vi "TemperatureCorrection.vi"(0 "Action":enum16{"Reset", "Calculate", "Correct"}(ring), 1 "Sensor Index":i32, 2 "Current IN":dbl[](array[numeric]), 3 "Actual temperature":dbl, 4 "Correction temperature":dbl format="%.2f") -> (5 "Current OUT":dbl[](array[numeric]), 6 "Correction factor":dbl)   [LabVIEW 2013]
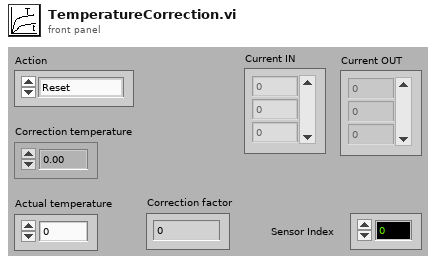
[diagram p1: front panel]
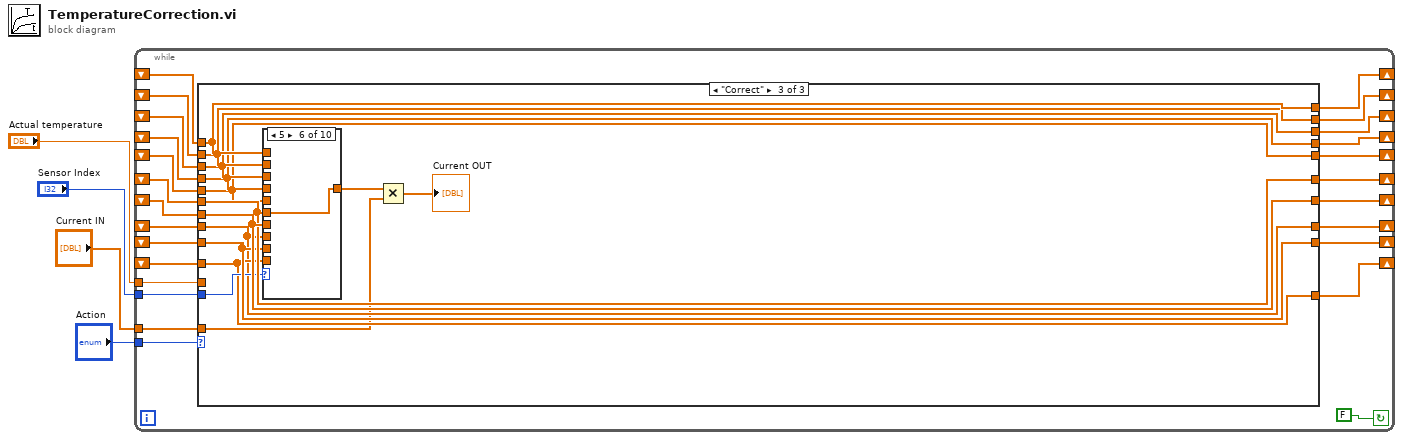
[diagram p0: block diagram]
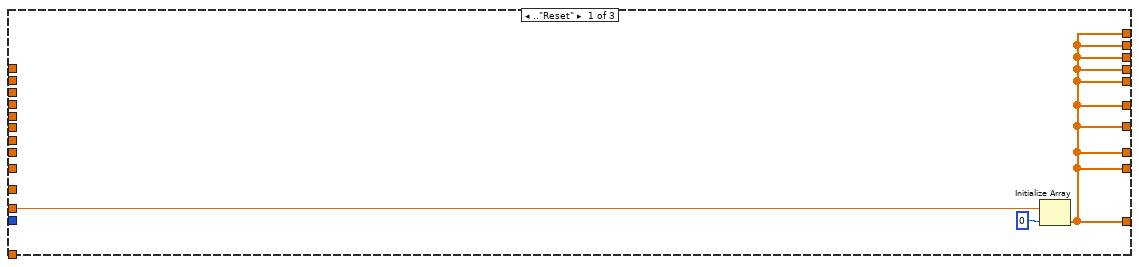
[diagram p2: hidden frame]
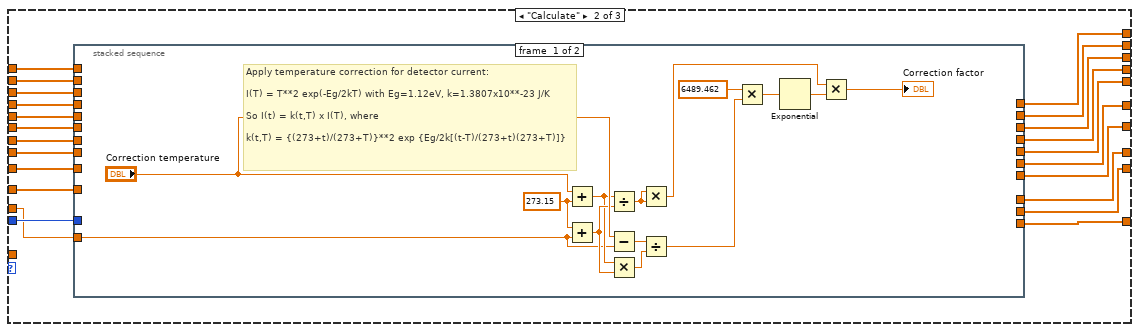
[diagram p3: hidden frame]
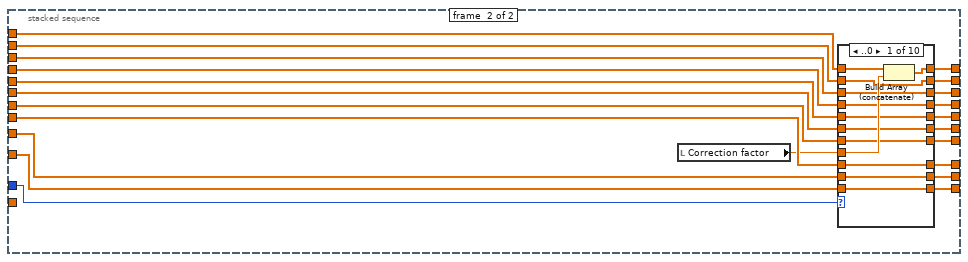
[diagram p4: hidden frame]
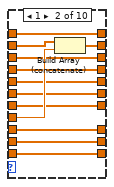
[diagram p5: hidden frame]
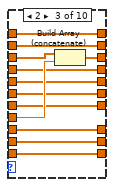
[diagram p6: hidden frame]
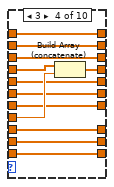
[diagram p7: hidden frame]
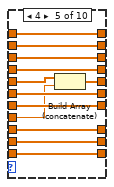
[diagram p8: hidden frame]
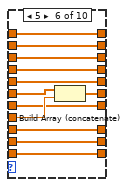
[diagram p9: hidden frame]
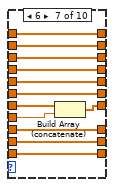
[diagram p10: hidden frame]
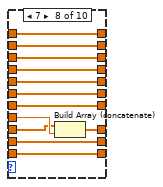
[diagram p11: hidden frame]
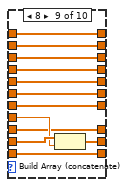
[diagram p12: hidden frame]
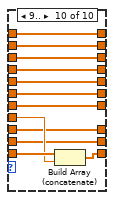
[diagram p13: hidden frame]
diagram:
  n1 = while {
    shift-left: _ -> [w10]
    shift-right: [w9] -> _
    tunnel: "Sensor Index" -> [w11]
    shift-left: _ -> [w12]
    shift-right: [w20] -> _
    shift-left: _ -> [w13]
    shift-right: [w8] -> _
    shift-left: _ -> [w14]
    shift-right: [w21] -> _
    shift-left: _ -> [w15]
    shift-right: [w22] -> _
    shift-left: _ -> [w16]
    shift-right: [w23] -> _
    shift-left: _ -> [w17]
    shift-right: [w24] -> _
    shift-left: _ -> [w18]
    shift-right: [w25] -> _
    shift-left: _ -> [w19]
    shift-right: [w26] -> _
    tunnel: "Actual temperature" -> [w28]
    shift-left: _ -> [w29]
    shift-right: [w27] -> _
    tunnel: "Current IN" -> [w6]
    tunnel: "Action" -> [w5]
    stop <- FALSE continue-if-true
    n2 = case shown="\"Correct\"" w5 {
      tunnel: [w32 w51 w224] -> w27
      tunnel: w29 -> [_ w53 w224]
      tunnel: w28 -> [w31 w52 _]
      tunnel: [w32 w49 w223] -> w26
      tunnel: [w32 w46 w222] -> w25
      tunnel: [w32 w45 w221] -> w24
      tunnel: [w32 w43 w220] -> w23
      tunnel: [w32 w42 w219] -> w22
      tunnel: [w32 w41 w218] -> w21
      tunnel: [w32 w40 w214] -> w8
      tunnel: [w32 w34 w217] -> w20
      tunnel: w19 -> [_ w50 w223]
      tunnel: w18 -> [_ w48 w222]
      tunnel: w17 -> [_ w47 w221]
      tunnel: w16 -> [_ w44 w220]
      tunnel: w15 -> [_ w39 w219]
      tunnel: w14 -> [_ w38 w218]
      tunnel: w13 -> [_ w37 w214]
      tunnel: w12 -> [_ w36 w217]
      tunnel: w11 -> [_ w54 w216]
      tunnel: w10 -> [_ w35 w215]
      tunnel: [w32 w33 w215] -> w9
      tunnel: w6 -> [_ _ w211]
      frame .."Reset" {
        n3 = Initialize Array(w31, 0) -> (w32:dbl[])
      }
      frame "Calculate" {
        n4 = stacked-sequence {
          tunnel: w54 -> [_ w90]
          tunnel: w53 -> [_ w89]
          tunnel: w52 -> [w55 _]
          tunnel: [_ w88] -> w51
          tunnel: w50 -> [_ w87]
          tunnel: [_ w86] -> w49
          tunnel: w48 -> [_ w85]
          tunnel: w47 -> [_ w84]
          tunnel: [_ w83] -> w46
          tunnel: [_ w82] -> w45
          tunnel: w44 -> [_ w81]
          tunnel: [_ w80] -> w43
          tunnel: [_ w79] -> w42
          tunnel: [_ w78] -> w41
          tunnel: [_ w77] -> w40
          tunnel: w39 -> [_ w76]
          tunnel: w38 -> [_ w75]
          tunnel: w37 -> [_ w74]
          tunnel: w36 -> [_ w73]
          tunnel: w35 -> [_ w72]
          tunnel: [_ w71] -> w34
          tunnel: [_ w70] -> w33
          frame #0 {
            w56 = 273.15
            # "Apply temperature correction for detector current:\n\nI(T) = T**2 exp(-Eg/2kT) with Eg=1.12eV, k=1.3807x10**-23 J/K\n\nSo I(t) = k(t,T) x I(T), where\n\nk(t,T) = {(273+t)/(273+T)}**2 exp {Eg/2k[(t-T)/(273+t)(273+T)]}"
            n5 = Add(x="Correction temperature", y=w56) -> (x+y=w58:dbl)
            n6 = Add(x=w56, y=w55) -> (x+y=w59:dbl)
            n7 = Divide(x=w58, y=w59) -> (x/y=w57:dbl)
            n8 = Subtract(x="Correction temperature", y=w55) -> (x-y=w61:dbl)
            n9 = Multiply(x=w58, y=w59) -> (x*y=w62:dbl)
            n10 = Multiply(x=w57, y=w57) -> (x*y=w65:dbl)
            n11 = Divide(x=w61, y=w62) -> (x/y=w64:dbl)
            n12 = Multiply(x=6489.462, y=w64) -> (x*y=w66:dbl)
            n13 = Exponential(1:w66) -> (0:w67:dbl)
            n14 = Multiply(x=w65, y=w67) -> (x*y=→"Correction factor":dbl)
          }
          frame #1 {
            n15 = local read "Correction factor"() -> (w69:dbl)
            n16 = case shown="..0" w90 {
              tunnel: w89 -> [w102 w111 w123 w135 w148 w159 w171 w183 w195 w207]
              tunnel: w69 -> [w101 w113 w126 w136 w139 w160 w174 w186 w197 w209]
              tunnel: [w100 w111 w123 w135 w148 w159 w171 w183 w195 w207] -> w88
              tunnel: w87 -> [w99 w114 w122 w134 w147 w158 w170 w182 w194 w206]
              tunnel: [w99 w112 w122 w134 w147 w158 w170 w182 w194 w206] -> w86
              tunnel: w85 -> [w98 w110 w125 w133 w146 w157 w169 w181 w193 w205]
              tunnel: w84 -> [w97 w109 w115 w138 w145 w156 w168 w180 w192 w204]
              tunnel: [w98 w110 w124 w133 w146 w157 w169 w181 w193 w205] -> w83
              tunnel: [w97 w109 w115 w137 w145 w156 w168 w180 w192 w204] -> w82
              tunnel: w81 -> [w96 w108 w116 w132 w144 w155 w173 w179 w191 w203]
              tunnel: [w96 w108 w116 w132 w144 w155 w172 w179 w191 w203] -> w80
              tunnel: [w95 w107 w117 w131 w143 w161 w167 w178 w190 w202] -> w79
              tunnel: w76 -> [w95 w107 w117 w131 w143 w162 w167 w178 w190 w202]
              tunnel: w75 -> [w94 w106 w118 w130 w150 w154 w166 w177 w189 w201]
              tunnel: [w94 w106 w118 w130 w149 w154 w166 w177 w189 w201] -> w78
              tunnel: [w93 w105 w119 w129 w142 w153 w165 w185 w188 w200] -> w77
              tunnel: w74 -> [w93 w105 w119 w129 w142 w153 w165 w184 w188 w200]
              tunnel: w73 -> [w92 w104 w120 w128 w141 w152 w164 w176 w198 w199]
              tunnel: w72 -> [w91 w103 w121 w127 w140 w151 w163 w175 w187 w210]
              tunnel: [w92 w104 w120 w128 w141 w152 w164 w176 w196 w199] -> w71
              tunnel: [w91 w103 w121 w127 w140 w151 w163 w175 w187 w208] -> w70
              frame ..0 {
                n17 = Build Array (concatenate)(w102, w101) -> (w100:dbl[])
              }
              frame 1 {
                n18 = Build Array (concatenate)(w114, w113) -> (w112:dbl[])
              }
              frame 2 {
                n19 = Build Array (concatenate)(w125, w126) -> (w124:dbl[])
              }
              frame 3 {
                n20 = Build Array (concatenate)(w138, w136) -> (w137:dbl[])
              }
              frame 4 {
                n21 = Build Array (concatenate)(w150, w139) -> (w149:dbl[])
              }
              frame 5 {
                n22 = Build Array (concatenate)(w162, w160) -> (w161:dbl[])
              }
              frame 6 {
                n23 = Build Array (concatenate)(w173, w174) -> (w172:dbl[])
              }
              frame 7 {
                n24 = Build Array (concatenate)(w184, w186) -> (w185:dbl[])
              }
              frame 8 {
                n25 = Build Array (concatenate)(w198, w197) -> (w196:dbl[])
              }
              frame 9.. {
                n26 = Build Array (concatenate)(w210, w209) -> (w208:dbl[])
              }
            }
          }
        }
      }
      frame "Correct" {
        n27 = case shown="5" w216 {
          tunnel: w224 -> [w225 _ _ _ _ _ _ _ _ _]
          tunnel: [w225 w226 w227 w228 w229 w230 w231 w232 w233 w234] -> w213
          tunnel: w223 -> [_ w226 _ _ _ _ _ _ _ _]
          tunnel: w222 -> [_ _ w227 _ _ _ _ _ _ _]
          tunnel: w221 -> [_ _ _ w228 _ _ _ _ _ _]
          tunnel: w220 -> [_ _ _ _ _ _ w231 _ _ _]
          tunnel: w219 -> [_ _ _ _ _ w230 _ _ _ _]
          tunnel: w218 -> [_ _ _ _ w229 _ _ _ _ _]
          tunnel: w214 -> [_ _ _ _ _ _ _ w232 _ _]
          tunnel: w217 -> [_ _ _ _ _ _ _ _ w233 _]
          tunnel: w215 -> [_ _ _ _ _ _ _ _ _ w234]
          frame ..0 {
          }
          frame 1 {
          }
          frame 2 {
          }
          frame 3 {
          }
          frame 4 {
          }
          frame 5 {
          }
          frame 6 {
          }
          frame 7 {
          }
          frame 8 {
          }
          frame 9.. {
          }
        }
        n28 = Multiply(x=w213, y=w211) -> (x*y=→"Current OUT":dbl[])
      }
    }
  }
